vi "5PassPack.vi"() -> ()   [LabVIEW 2022 SP3]
panel:
  out "size(s) 2":i32[](array[numeric])
  out "2-D data array 2":i8[](array[numeric])
  out "size(s)":i32[](array[numeric])
  in  "2-D data array":i8[][][](array[numeric])
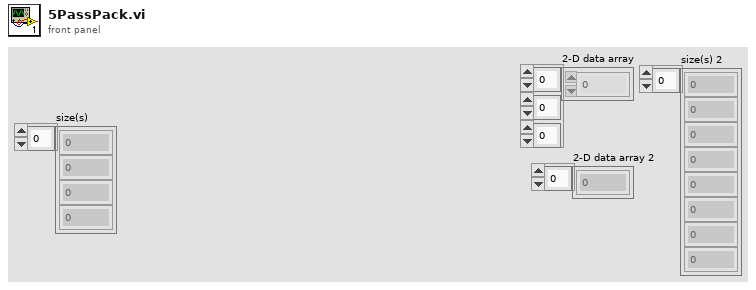
[diagram p1: front panel]
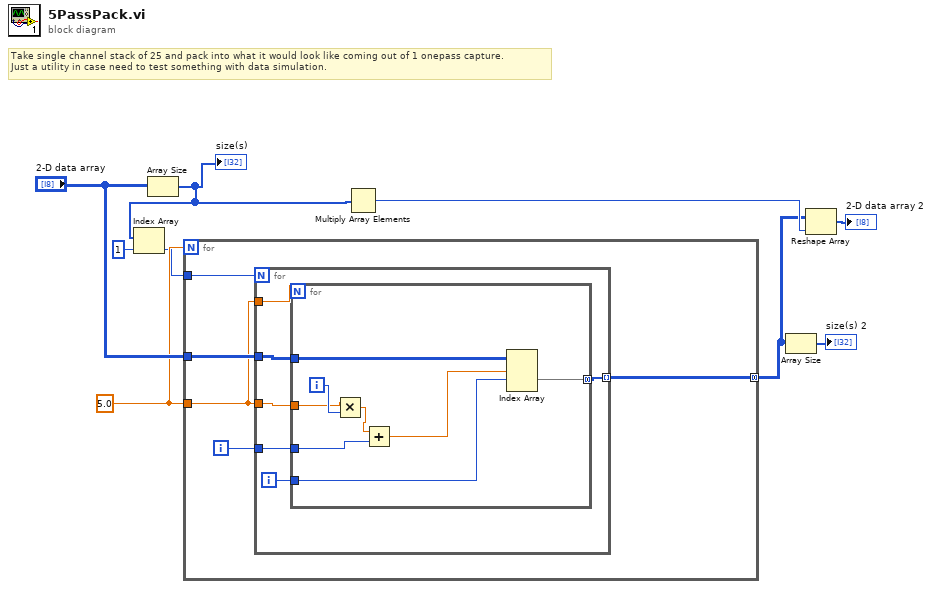
[diagram p0: block diagram]
diagram:
  w7 = 5.0 ("x")
  # "Take single channel stack of 25 and pack into what it would look like coming out of 1 onepass capture.\nJust a utility in case need to test something with data simulation."
  n1 = Array Size(array="2-D data array") -> (size(s)=w5:i32[])
  "size(s)" <- w5
  n2 = Index Array(array=w5, index=1) -> (element=w6:i32)
  n3 = for {
    N: w7 -> [_]
    tunnel: "2-D data array" -> [w14]
    tunnel: w7 -> [w10]
    tunnel: [w12] -> w2 mode=concatenating
    tunnel: w6 -> [w11]
    i -> [w13]
    n4 = for {
      N: w11 -> [_]
      tunnel: w14 -> [w20]
      tunnel: w13 -> [w16]
      tunnel: w10 -> [w19]
      tunnel: w10 -> [w18]
      tunnel: [w17] -> w12 mode=indexing
      i -> [w15]
      n5 = for {
        N: w19 -> [_]
        tunnel: w20 -> [w28]
        tunnel: w15 -> [w26]
        tunnel: w18 -> [w25]
        tunnel: [w22] -> w17 mode=concatenating
        tunnel: w16 -> [w21]
        i -> [w27]
        n6 = Multiply(x=w25, y=w27) -> (x*y=w24:dbl)
        n7 = Add(x=w24, y=w21) -> (x+y=w23:dbl)
        n8 = Index Array(array=w28, index (dim 0)=w23, index (dim 1)=w26) -> (element=w22:i8[])  [unwired: 1 in]
      }
    }
  }
  n9 = Multiply Array Elements(1:w5) -> (0:w4:i32)
  n10 = Array Size(array=w2) -> (size(s)=→"size(s) 2":i32[])
  n11 = Reshape Array(w2, w4) -> (→"2-D data array 2":i8[])
